vi "Add User Channel Folder.vi"(7 "Overwrite Existing?":bool=TRUE, 8 "error in (no error)":errorcluster, 9 "User Channel Folder Settings":T1, 10 "Base Node Path":string, 11 "SysDef Ref":T2) -> (0 "error out":errorcluster, 2 "New Node Path":string, 3 "SysDef Ref Out":T2)   [LabVIEW 2019, in "Simple SysDef API.lvlib"]
uses:
  <userlib>/SimpleSysDef/Simple SysDef API.lvlib
  <userlib>/SimpleSysDef/_SubVIs/System Definition Reference.ctl
  NationalInstruments.VeriStand.SystemDefinitionAPI
  <userlib>/SimpleSysDef/_SubVIs/Add Folder_Settings.ctl
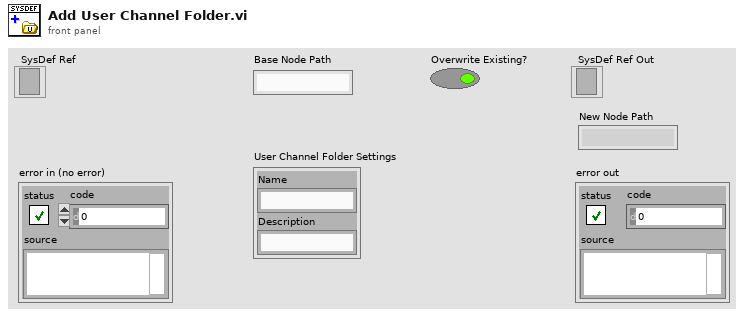
[diagram p1: front panel]
types:
  T1 = typedef "Simple SysDef API.lvlib/Add Folder_Settings.ctl" = cluster{"Name":string, "Description":string}
  T2 = typedef "Simple SysDef API.lvlib/System Definition Reference.ctl" = refnum<k24>
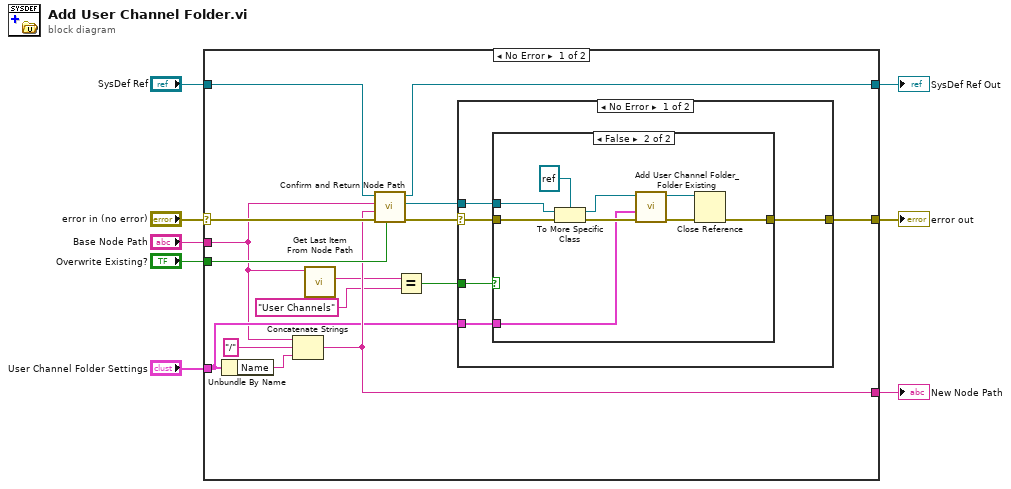
[diagram p0: block diagram]
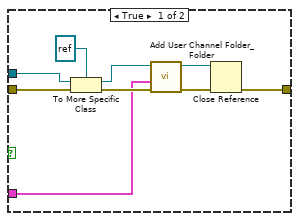
[diagram p2: hidden frame]
diagram:
  n1 = case shown="No Error" "error in (no error)" {
    selector: "error in (no error)" -> [w23 w49]
    tunnel: [w18 w49] -> w7
    tunnel: "SysDef Ref" -> [w22 w48]
    tunnel: [w21 w48] -> w5
    tunnel: "Base Node Path" -> [w12 _]
    tunnel: "Overwrite Existing?" -> [w15 _]
    tunnel: "User Channel Folder Settings" -> [w13 _]
    tunnel: [w14 _] -> w1
    frame No Error {
      n2 = Unbundle By Name(w13) -> ("Name"=w19:string)
      n3 = Concatenate Strings(w12, "/" ("string"), w19) -> (w14:string)
      n4 = call <userlib>:"Get Last Item From Node Path.vi"("Name"=w12) -> ("Last Item"=w11:string)  [unwired: 9 in, 1 out]
      n5 = call <userlib>:"Confirm and Return Node Path.vi"("Overwrite Existing?"=w15, "error in (no error)"=w23, "New Node Path"=w14, "Base Node Path"=w12, "SysDef Ref"=w22) -> ("error out"=w16:errorcluster, "Node Ref"=w17:refnum<k24>, "SysDef Ref Out"=w21:T2)  [unwired: 4 in]
      n6 = Equal?(x=w11, y="User Channels") -> (x = y?=w9:bool)
      n7 = case shown="No Error" w16 {
        selector: w16 -> [w27 w47]
        tunnel: [w26 w47] -> w18
        tunnel: w17 -> [w28 _]
        tunnel: w13 -> [w25 _]
        tunnel: w9 -> [w24 _]
        frame No Error {
          n8 = case shown="False" w24 {
            tunnel: w28 -> [w37 w46]
            tunnel: w27 -> [w36 w45]
            tunnel: [w35 w44] -> w26
            tunnel: w25 -> [w29 w38]
            frame True {
              n9 = To More Specific Class(target class=refnum<k24> refnum ("Node Ref"), reference=w37, error in=w36) -> (specific class reference=w33:refnum<k24>, error out=w32:errorcluster)
              n10 = call <userlib>:"Add User Channel Folder_Folder.vi"("error in (no error)"=w32, "User Channel Folder Settings"=w29, "User Channels Ref"=w33) -> ("error out"=w31:errorcluster, "User Channels Ref out"=w30:refnum<k24>)  [unwired: 7 in]
              n11 = Close Reference(reference=w30, error in (no error)=w31) -> (error out=w35:errorcluster)
            }
            frame False {
              n12 = To More Specific Class(target class=refnum<k24> refnum ("Node Ref"), reference=w46, error in=w45) -> (specific class reference=w39:refnum<k24>, error out=w42:errorcluster)
              n13 = call <userlib>:"Add User Channel Folder_Folder Existing.vi"("error in (no error)"=w42, "User Channel Folder Settings"=w38, "User Channels Ref"=w39) -> ("error out"=w41:errorcluster, "User Channels Ref out"=w40:refnum<k24>)  [unwired: 7 in]
              n14 = Close Reference(reference=w40, error in (no error)=w41) -> (error out=w44:errorcluster)
            }
          }
        }
        frame Error {
        }
      }
    }
    frame Error {
    }
  }
  "SysDef Ref Out" <- w5
  "error out" <- w7
  "New Node Path" <- w1
